vi "PSPOP_Demo Registration.vi"(7 "Name":string, 8 "error in (no error)":errorcluster, 11 "Signal Settings ref":refnum<vi>) -> (0 "error out":errorcluster)   [LabVIEW 2016]
doc: "VI to hold all the different type registrations for this specific demo.\n\nType Sensitive Popup \nCopyright © 2007, J. David Saunders\nAll rights reserved."
uses:
  Private/Ctrls/POP_Popup Call Parameters.ctl
  Private/Ctrls/POP_Data Type.ctl
  <vilib>/Utility/miscctls.llb/LVBrowseOptionsTypeDef.ctl
panel:
  in  "Show Popup (type only)":T1={"Prop Type"=enum."Unkown", "Initial Value"=variant, "Caption Strings"=[], "Ring Strings"=[], "Cell Rect"={"left"=0, "top"=0, "right"=0, "bottom"=0}, "Mouse Coords"={"x"=0, "y"=0}, "Call Data"=variant, "Ring Values"=[], "Browse Options"={"Prompt"="", "Match Pattern"="", "Mode"=enum."existing file", "Start Path"=path "", "Pattern Label"="", "Button Text"=""}, "Combo Box"={"Allow Undefined Strings"=FALSE}}
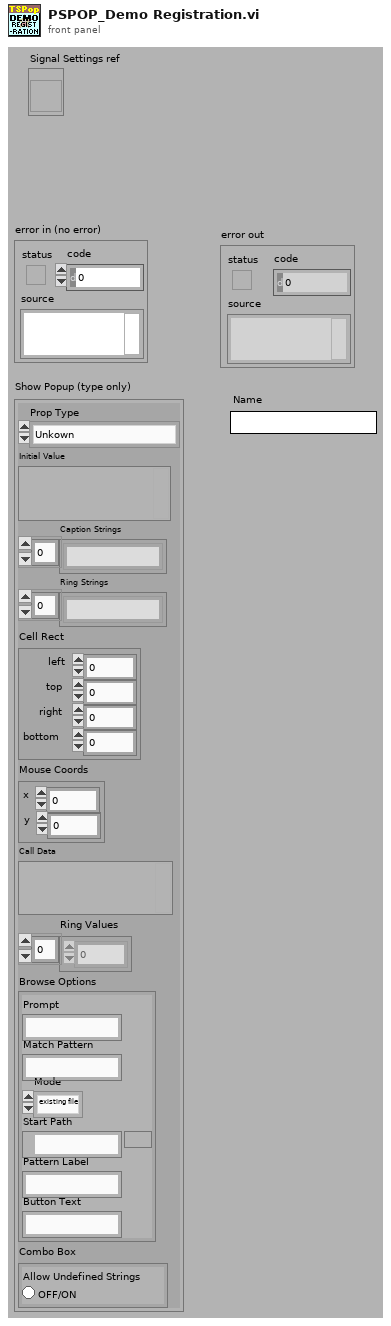
[diagram p1: front panel]
types:
  T1 = typedef "POP_Popup Call Parameters.ctl" = cluster{"Prop Type":T2, "Initial Value":variant, "Caption Strings":string[], "Ring Strings":string[], "Cell Rect":cluster{"left":i16, "top":i16, "right":i16, "bottom":i16}, "Mouse Coords":cluster{"x":i16, "y":i16}, "Call Data":variant, "Ring Values":ext[], "Browse Options":T3, "Combo Box":cluster{"Allow Undefined Strings":bool}}
  T2 = typedef "POP_Data Type.ctl" = enum16{"NO POPUP", "Unkown", "String", "Integer", "Float", "Color", "Boolean", "Ring", "Captioned String", "Captioned Integer", "Button Color", "2 Int Cluster", "4 Int Cluster", "6-Dbl Cluster", "Path", "Combox", "Time", "ShotCut String"}
  T3 = typedef "LVBrowseOptionsTypeDef.ctl" = cluster{"Prompt":string, "Match Pattern":string, "Mode":enum32{"existing file", "new file", "new or existing file", "existing dir", "new dir", "new or existing dir", "existing file (use LLBs)", "new file (use LLBs)", "new or existing file (use LLBs)", "new or existing file or directory (use LLBs)", "existing dir (use LLBs)", "new dir (use LLBs)", "new or existing dir (use LLBs)", "existing file or dir", "new file or dir", "new or existing file or dir", "existing file or dir (use LLBs)", "new file or dir (use LLBs)"}, "Start Path":path, "Pattern Label":string, "Button Text":string}
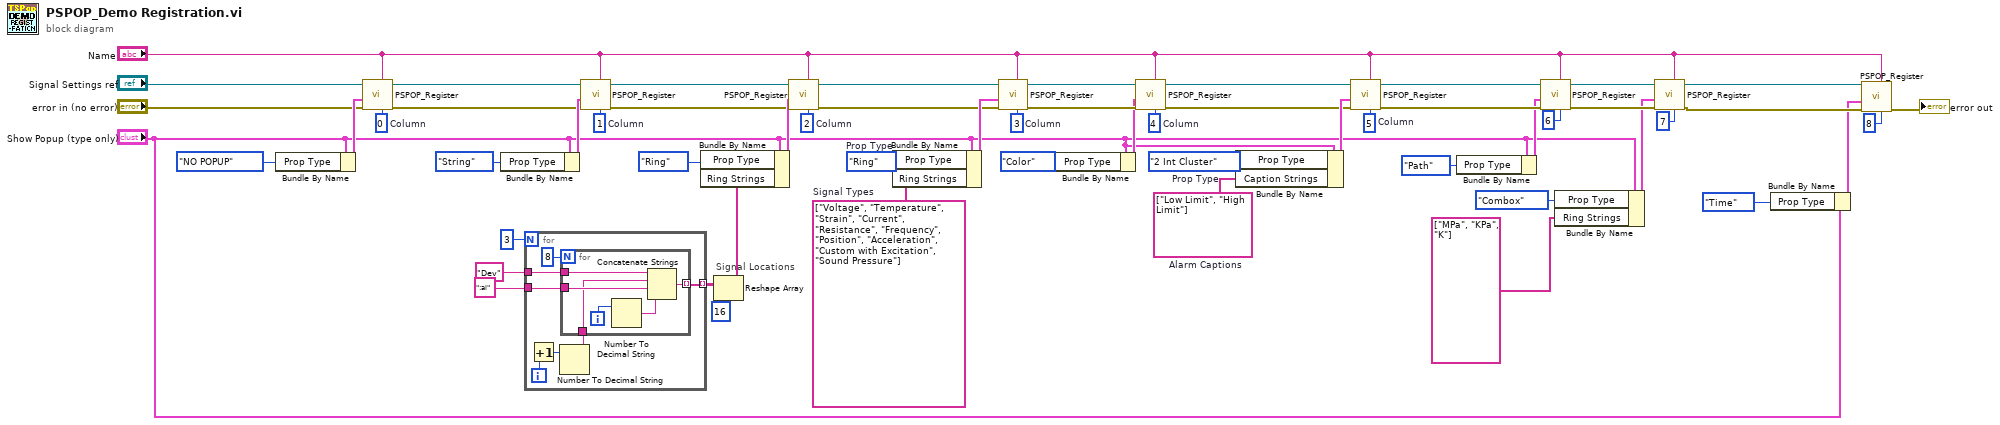
[diagram p0: block diagram]
diagram:
  w26 = 0  # Column
  w27 = 5  # Column
  w32 = POP_Data_Type."2 Int Cluster"  # Prop Type
  w38 = 4  # Column
  w45 = 2  # Column
  w46 = 1  # Column
  w50 = 3  # Column
  w52 = POP_Data_Type."Ring"  # Prop Type
  w49 = string[] ["Voltage", "Temperature", "Strain", "Current", "Resistance", "Frequency", "Position", "Acceleration", "Custom with Excitation", "Sound Pressure"]  # Signal Types
  w31 = string[] ["Low Limit", "High Limit"]  # Alarm Captions
  # "Signal Locations"
  n1 = Bundle By Name(cluster="Show Popup (type only)", "Prop Type"=POP_Data_Type."NO POPUP") -> (w21:T1)
  n2 = call "PSPOP_Register.vi"("Col (unwired = all columns)"=w26, "Name"="Name", "error in (no error)"="error in (no error)", "Parameters"=w21, "Ctl Refnum"="Signal Settings ref") -> ("error out"=w24:errorcluster, "dup ref out"=w25:refnum<vi>)  [unwired: 5 in]
  n3 = Bundle By Name(cluster="Show Popup (type only)", "Prop Type"=POP_Data_Type."String") -> (w47:T1)
  n4 = for {
    N: 3 -> [_]
    tunnel: "Dev" -> [w61]
    tunnel: ":ai" -> [w60]
    tunnel: [w58] -> w54 mode=indexing
    i -> [w63]
    n5 = Increment(x=w63) -> (x+1=w62:i32)
    n6 = Number To Decimal String(number=w62) -> (decimal integer string=w59:string)  [unwired: 1 in]
    n7 = for {
      N: 8 -> [_]
      tunnel: w61 -> [w69]
      tunnel: w60 -> [w68]
      tunnel: w59 -> [w67]
      tunnel: [w65] -> w58 mode=indexing
      i -> [w70]
      n8 = Number To Decimal String(number=w70) -> (decimal integer string=w66:string)  [unwired: 1 in]
      n9 = Concatenate Strings(w69, w67, w68, w66) -> (w65:string)
    }
  }
  n10 = call "PSPOP_Register.vi"("Col (unwired = all columns)"=w46, "Name"="Name", "error in (no error)"=w24, "Parameters"=w47, "Ctl Refnum"=w25) -> ("error out"=w41:errorcluster, "dup ref out"=w42:refnum<vi>)  [unwired: 5 in]
  n11 = Reshape Array(w54, 16 ("dimension size")) -> (w40:string[])
  n12 = Bundle By Name(cluster="Show Popup (type only)", "Prop Type"=POP_Data_Type."Ring", "Ring Strings"=w40) -> (w43:T1)
  n13 = call "PSPOP_Register.vi"("Col (unwired = all columns)"=w45, "Name"="Name", "error in (no error)"=w41, "Parameters"=w43, "Ctl Refnum"=w42) -> ("error out"=w36:errorcluster, "dup ref out"=w37:refnum<vi>)  [unwired: 5 in]
  n14 = Bundle By Name(cluster="Show Popup (type only)", "Prop Type"=w52, "Ring Strings"=w49) -> (w51:T1)
  n15 = call "PSPOP_Register.vi"("Col (unwired = all columns)"=w50, "Name"="Name", "error in (no error)"=w36, "Parameters"=w51, "Ctl Refnum"=w37) -> ("error out"=w35:errorcluster, "dup ref out"=w34:refnum<vi>)  [unwired: 5 in]
  n16 = Bundle By Name(cluster="Show Popup (type only)", "Prop Type"=POP_Data_Type."Color") -> (w33:T1)
  n17 = call "PSPOP_Register.vi"("Col (unwired = all columns)"=w38, "Name"="Name", "error in (no error)"=w35, "Parameters"=w33, "Ctl Refnum"=w34) -> ("error out"=w28:errorcluster, "dup ref out"=w29:refnum<vi>)  [unwired: 5 in]
  n18 = Bundle By Name(cluster="Show Popup (type only)", "Prop Type"=w32, "Caption Strings"=w31) -> (w30:T1)
  n19 = call "PSPOP_Register.vi"("Col (unwired = all columns)"=w27, "Name"="Name", "error in (no error)"=w28, "Parameters"=w30, "Ctl Refnum"=w29) -> ("error out"=w18:errorcluster, "dup ref out"=w19:refnum<vi>)  [unwired: 5 in]
  n20 = Bundle By Name(cluster="Show Popup (type only)", "Prop Type"=POP_Data_Type."Path") -> (w16:T1)
  n21 = call "PSPOP_Register.vi"("Col (unwired = all columns)"=6, "Name"="Name", "error in (no error)"=w18, "Parameters"=w16, "Ctl Refnum"=w19) -> ("error out"=w12:errorcluster, "dup ref out"=w13:refnum<vi>)  [unwired: 5 in]
  n22 = Bundle By Name(cluster="Show Popup (type only)", "Prop Type"=POP_Data_Type."Combox", "Ring Strings"=string[] ["MPa", "KPa", "K"]) -> (w10:T1)
  n23 = call "PSPOP_Register.vi"("Col (unwired = all columns)"=7, "Name"="Name", "error in (no error)"=w12, "Parameters"=w10, "Ctl Refnum"=w13) -> ("error out"=w5:errorcluster, "dup ref out"=w6:refnum<vi>)  [unwired: 5 in]
  n24 = Bundle By Name(cluster="Show Popup (type only)", "Prop Type"=POP_Data_Type."Time") -> (w3:T1)
  n25 = call "PSPOP_Register.vi"("Col (unwired = all columns)"=8, "Name"="Name", "error in (no error)"=w5, "Parameters"=w3, "Ctl Refnum"=w6) -> ("error out"=→"error out":errorcluster)  [unwired: 5 in, 1 out]
